vi "getGratingWheelStatus.vi"(0 "SpectrographClientCommunicator in":refnum<class "SpectrographClientCommunicator.lvclass">, 11 "error in (no error)":errorcluster) -> (4 "SpectrographClientCommunicator out":refnum<class "SpectrographClientCommunicator.lvclass">, 6 "Status":string, 8 "Current Position":string, 10 "Error Code":string, 15 "error out":errorcluster)   [LabVIEW 2016, in "SpectrographClientCommunicator.lvclass"]
uses:
  SpectrographClientCommunicator.lvclass
  SpectrographTypeDef/SpectrographCMDs.ctl
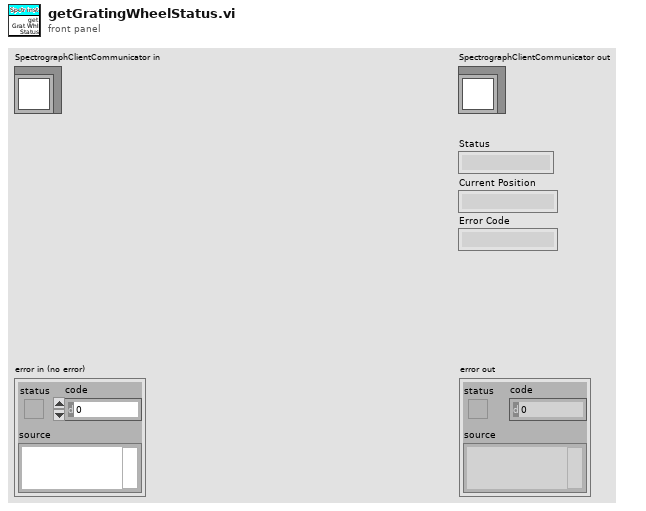
[diagram p1: front panel]
types:
  T1 = typedef "SpectrographCMDs.ctl" = enum16{"getFilterWheelPosition", "getGratingWheelPosition", "moveLinearStage", "moveGratingWheel", "moveFilterWheel", "homeLinearStage", "getLinearStageStatus", "getGratingWheelStatus", "getFilterWheelStatus", "stopAllMotion"}
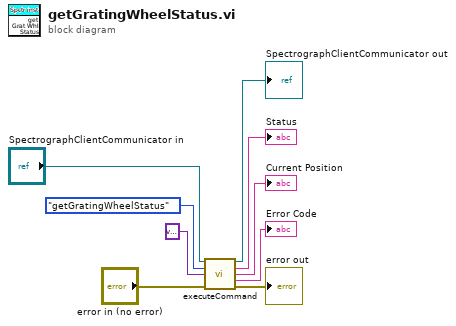
[diagram p0: block diagram]
diagram:
  n1 = call "executeCommand.vi"("SpectrographClientCommunicator in"="SpectrographClientCommunicator in", "Command"=SpectrographCMDs."getGratingWheelStatus", "input"=variant, "error in (no error)"="error in (no error)") -> ("SpectrographClientCommunicator out"=→"SpectrographClientCommunicator out":refnum<class "SpectrographClientCommunicator.lvclass">, "Status"=→"Status":string, "Current Position"=→"Current Position":string, "Error Code"=→"Error Code":string, "error out"=→"error out":errorcluster)  [unwired: 7 in]
